vi "Sha-1 Extend to 80 Words.vi"(11 "16 32-bit Words In":u32[](array[numeric])) -> (3 "80 32 Bit Words Out":u32[](array[numeric]))   [LabVIEW 2014]
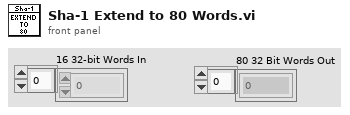
[diagram p1: front panel]
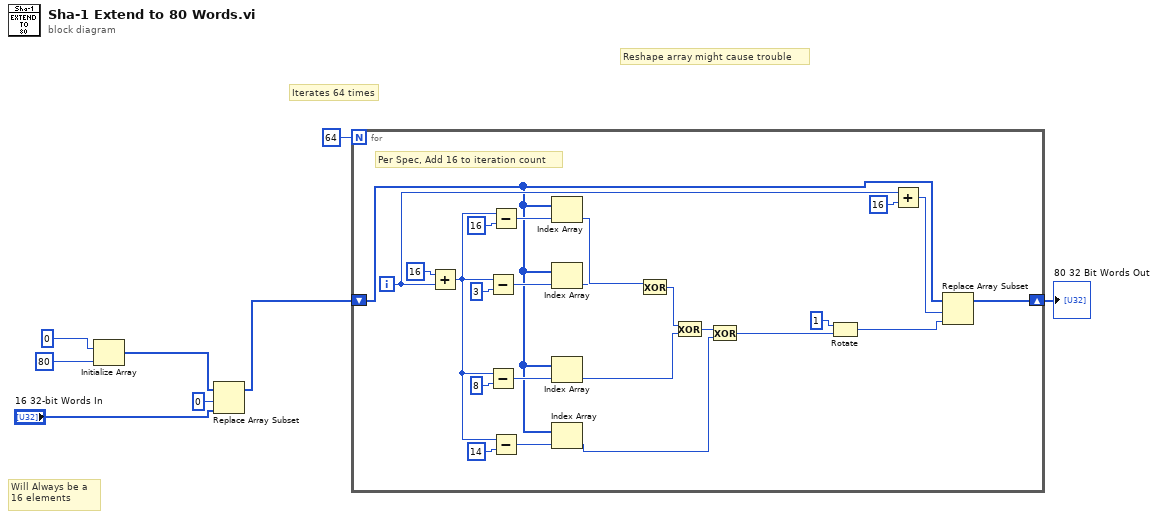
[diagram p0: block diagram]
diagram:
  # "Will Always be a \n16 elements"
  # "Reshape array might cause trouble"
  # "Iterates 64 times"
  n1 = Initialize Array(u32 0 ("dimension size"), 80 ("dimension size")) -> (w5:u32[])
  n2 = Replace Array Subset(array=w5, new element="16 32-bit Words In", index=0) -> (w2:u32[])
  n3 = for {
    N: 64 -> [_]
    shift-right: [w17] -> w1
    shift-left: w2 -> [w16]
    i -> [w20]
    # "Per Spec, Add 16 to iteration count"
    n4 = Add(x=16, y=w20) -> (x+y=w31:i32)
    n5 = Subtract(x=w31, y=3 ("length")) -> (x-y=w23:i32)
    n6 = Subtract(x=w31, y=8 ("length")) -> (x-y=w24:i32)
    n7 = Subtract(x=w31, y=16 ("length")) -> (x-y=w26:i32)
    n8 = Subtract(x=w31, y=14 ("length")) -> (x-y=w25:i32)
    n9 = Index Array(array=w16, index=w26) -> (element=w14:u32)
    n10 = Index Array(array=w16, index=w23) -> (element=w13:u32)
    n11 = Index Array(array=w16, index=w24) -> (element=w12:u32)
    n12 = Index Array(array=w16, index=w25) -> (element=w11:u32)
    n13 = Exclusive Or(1:w13, 2:w14) -> (0:w22:u32)
    n14 = Exclusive Or(1:w12, 2:w22) -> (0:w21:u32)
    n15 = Exclusive Or(1:w11, 2:w21) -> (0:w10:u32)
    n16 = Rotate(1:w10, 2:i16 1 ("y")) -> (0:w9:u32)
    n17 = Add(x=w20, y=16 ("x")) -> (x+y=w18:i32)
    n18 = Replace Array Subset(array=w16, new element=w9, index=w18) -> (w17:u32[])
  }
  "80 32 Bit Words Out" <- w1
